vi "Register Window.vi"(8 "error in (no error)":errorcluster, 11 "Window Name":string) -> (0 "error out":errorcluster)   [LabVIEW 2020, in "Group Interface.lvlib"]
uses:
  Group Interface.lvlib
  3e5b46f5-ff7f-4059-b27c-edcccd9e1d79.vi
  <userlib>/_NEVSTOP/Communicable State Machine(CSM)/addons/API-String-Arugments-Support/_Support/Data To API String Arguments.vi
  <userlib>/_NEVSTOP/Communicable State Machine(CSM)/Communicable State Machine.lvlib
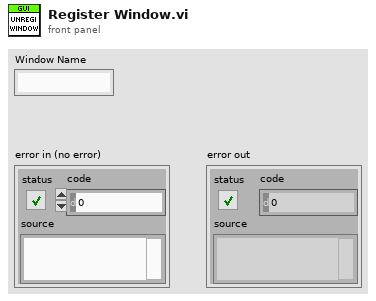
[diagram p1: front panel]
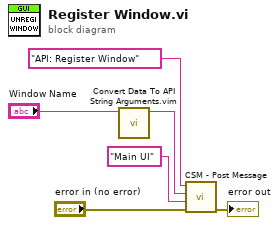
[diagram p0: block diagram]
diagram:
  n1 = call "Convert Data To API String Arguments.vim"("Data"="Window Name") -> ("API String"=w4:string)  [unwired: 7 in, 1 out]
  n2 = call <userlib>:"CSM - Post Message.vi"("Error In (No Error)"="error in (no error)", "Target Module"="Main UI", "Arguments (\"\")"=w4, "State"="API: Register Window") -> ("error out"=→"error out":errorcluster)  [unwired: 7 in]
